vi "libssh2_channel_get_exit_signal.vi"(8 "error in (no error)":errorcluster, 11 "channel":T1) -> (0 "error out":errorcluster, 1 "errmsg":string, 2 "exitsignal":string, 4 "langtag":string)   [LabVIEW 2013, in "libssh2.lvlib"]
doc: "Gets the exit signal send by the process running on the remote host at the end of the named channel. Note that the exit signal may not be available if the process is still running on the remote host."
uses:
  libssh2.lvlib
  Channel Refnum.ctl
  Not A Channel.vi
  <vilib>/Utility/error.llb/Error Cluster From Error Code.vi
  Global Settings.vi
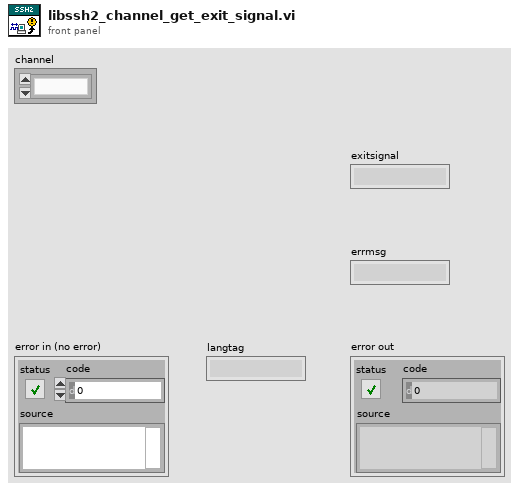
[diagram p1: front panel]
types:
  T1 = typedef "libssh2.lvlib/Channel Refnum.ctl" = refnum<k1>
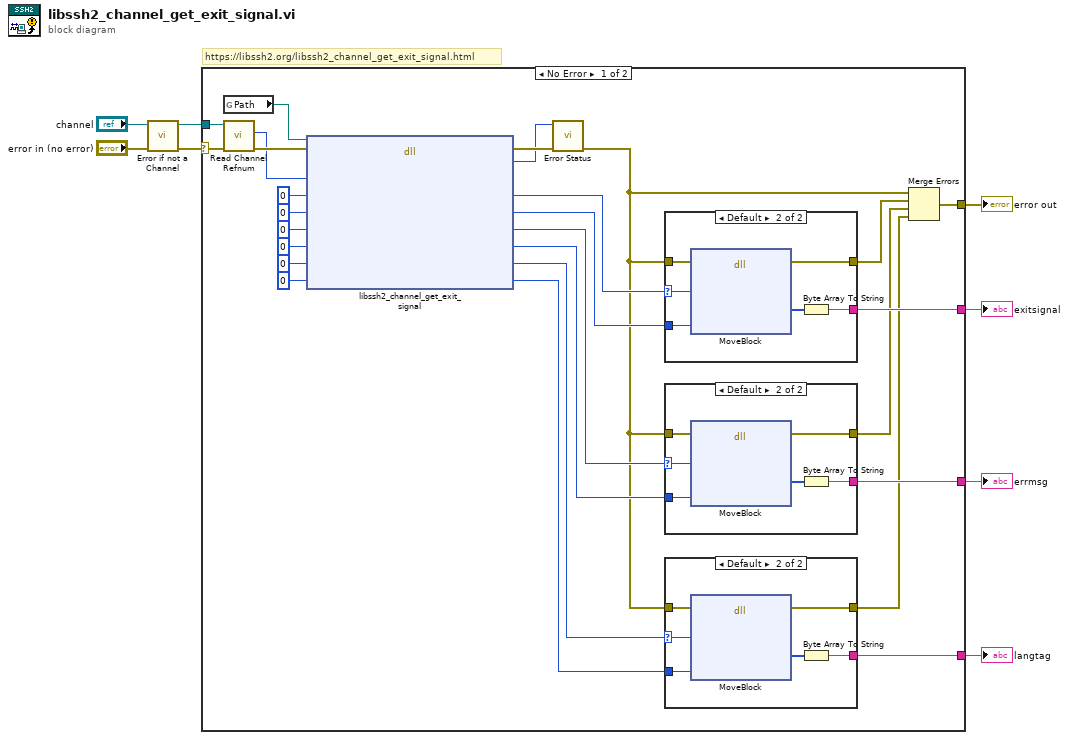
[diagram p0: block diagram]
diagram:
  # "https://libssh2.org/libssh2_channel_get_exit_signal.html"
  n1 = call "Error if not a Channel.vi"("error in (no error)"="error in (no error)", "channel"="channel") -> ("error out"=w3:errorcluster, "channel out"=w1:T1)  [unwired: 8 in]
  n2 = case shown="No Error" w3 {
    selector: w3 -> [w12 w57]
    tunnel: [w32 _] -> w8
    tunnel: w1 -> [w25 _]
    tunnel: [w23 w57] -> w7
    tunnel: [w19 _] -> w6
    tunnel: [w14 _] -> w5
    frame No Error {
      n3 = global read "Global Settings.vi" "Path"() -> (w11:path)
      n4 = call "Read Channel Refnum.vi"("error in (no error)"=w12, "channel"=w25) -> ("error out"=w27:errorcluster, "LIBSSH2_CHANNEL*"=w26:u64)  [unwired: 8 in]
      n5 = dll-call lib="C:/Users/pasca/source/repos/libssh2-labview/libssh2/libssh2**.*" fn="libssh2_channel_get_exit_signal"(path in=w11, error in=w27, "channel"=w26, "exitsignal"=u64 0, "exitsignal_len"=i64 0, "errmsg"=u64 0, "errmsg_len"=i64 0, "langtag"=u64 0, "langtag_len"=i64 0) -> (error out=w17:errorcluster, "return value"=w9:i32, "exitsignal"=w22:u64, "exitsignal_len"=w31:i64, "errmsg"=w21:u64, "errmsg_len"=w20:i64, "langtag"=w16:u64, "langtag_len"=w15:i64)  [unwired: 2 in, 1 out]
      n6 = call "Error Status.vi"("error in (no error)"=w17, "return value"=w9) -> ("error out"=w10:errorcluster)  [unwired: 8 in, 1 out]
      n7 = case shown="Default" w22 {
        selector: w22 -> [_ w51]
        tunnel: [_ w55] -> w32
        tunnel: w31 -> [_ w54]
        tunnel: [w50 w53] -> w24
        tunnel: w10 -> [w50 w52]
        frame 0 {
        }
        frame Default {
          n8 = dll-call lib="LabVIEW" fn="MoveBlock"(error in=w52, "ps"=w51, "size"=w54) -> (error out=w53:errorcluster, "pd"=w56:u8[])  [unwired: 6 in, 1 out]
          n9 = Byte Array To String(unsigned byte array=w56) -> (string=w55:string)
        }
      }
      n10 = case shown="Default" w21 {
        selector: w21 -> [_ w44]
        tunnel: [_ w48] -> w19
        tunnel: w20 -> [_ w47]
        tunnel: [w43 w46] -> w18
        tunnel: w10 -> [w43 w45]
        frame 0 {
        }
        frame Default {
          n11 = dll-call lib="LabVIEW" fn="MoveBlock"(error in=w45, "ps"=w44, "size"=w47) -> (error out=w46:errorcluster, "pd"=w49:u8[])  [unwired: 6 in, 1 out]
          n12 = Byte Array To String(unsigned byte array=w49) -> (string=w48:string)
        }
      }
      n13 = case shown="Default" w16 {
        selector: w16 -> [_ w37]
        tunnel: [_ w41] -> w14
        tunnel: w15 -> [_ w40]
        tunnel: [w36 w39] -> w13
        tunnel: w10 -> [w36 w38]
        frame 0 {
        }
        frame Default {
          n14 = dll-call lib="LabVIEW" fn="MoveBlock"(error in=w38, "ps"=w37, "size"=w40) -> (error out=w39:errorcluster, "pd"=w42:u8[])  [unwired: 6 in, 1 out]
          n15 = Byte Array To String(unsigned byte array=w42) -> (string=w41:string)
        }
      }
      n16 = Merge Errors(w10, w24, w18, w13) -> (w23:errorcluster)
    }
    frame Error {
    }
  }
  "error out" <- w7
  "exitsignal" <- w8
  "errmsg" <- w6
  "langtag" <- w5
